vi "S2C_STEP_ShowMenu.vi"(8 "Error In":errorcluster, 9 "Cell Position":T1, 10 "MenuRef":refnum<k9>, 11 "CtlRef":refnum<vi>) -> (0 "Error Out":errorcluster, 3 "Discard?":bool)   [LabVIEW 2015]
doc: "Loads the popup menu for the selected Fornax command parameter."
uses:
  <vilib>/Utility/miscctls.llb/LVRowAndColumnTypeDef.ctl
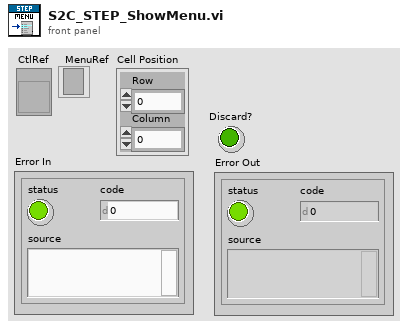
[diagram p1: front panel]
types:
  T1 = typedef "LVRowAndColumnTypeDef.ctl" = cluster{"Row":i32, "Column":i32}
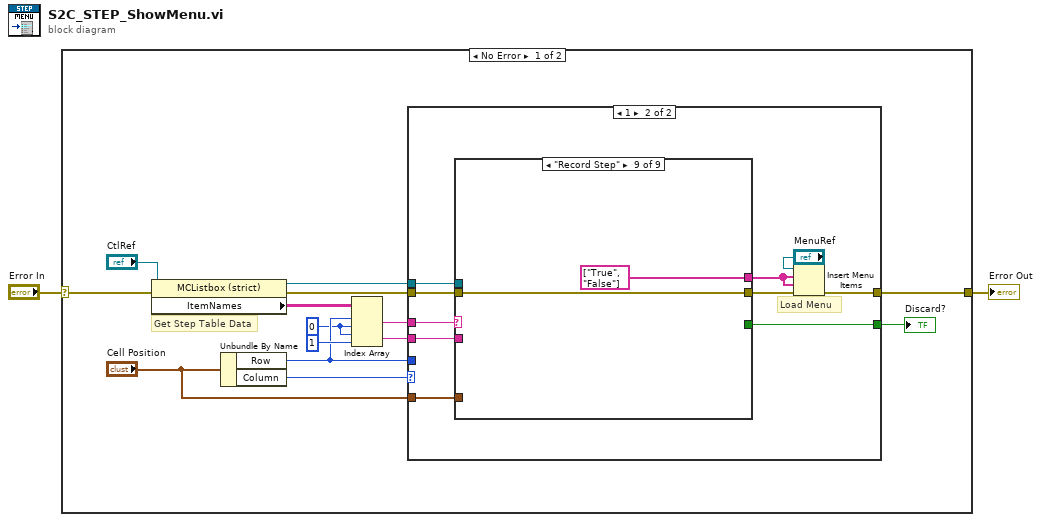
[diagram p0: block diagram]
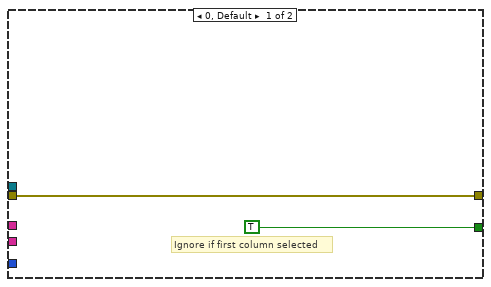
[diagram p2: hidden frame]
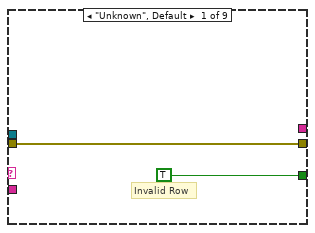
[diagram p3: hidden frame]
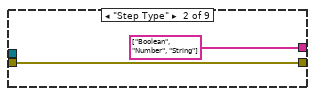
[diagram p4: hidden frame]
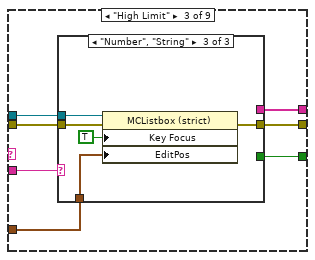
[diagram p5: hidden frame]
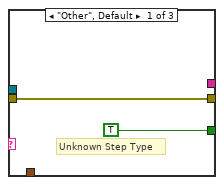
[diagram p6: hidden frame]
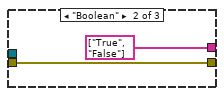
[diagram p7: hidden frame]
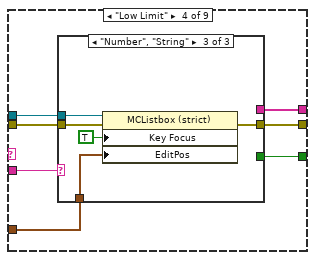
[diagram p8: hidden frame]
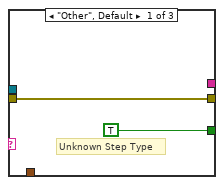
[diagram p9: hidden frame]
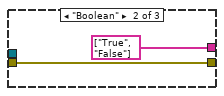
[diagram p10: hidden frame]
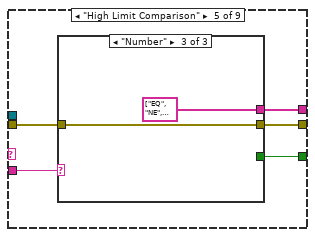
[diagram p11: hidden frame]
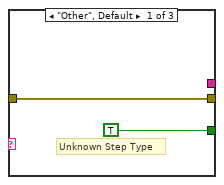
[diagram p12: hidden frame]
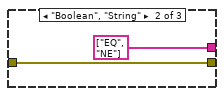
[diagram p13: hidden frame]
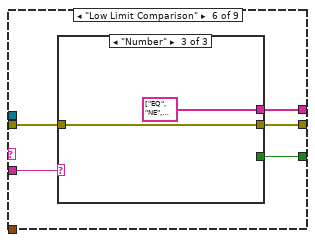
[diagram p14: hidden frame]
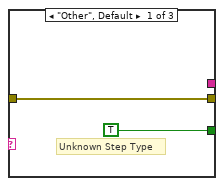
[diagram p15: hidden frame]
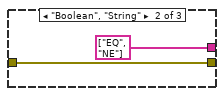
[diagram p16: hidden frame]
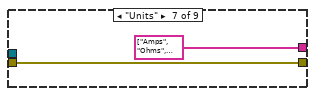
[diagram p17: hidden frame]
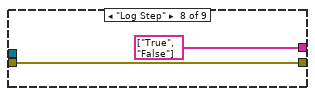
[diagram p18: hidden frame]
diagram:
  n1 = case shown="No Error" "Error In" {
    selector: "Error In" -> [w11 w93]
    tunnel: [w16 w93] -> w1
    frame No Error {
      w3 = 0 ("disabled index (col)")
      # "Get Step Table Data"
      n2 = property class="MCListbox (strict)"(reference="CtlRef", error in=w11) -> (reference out=w8:refnum<vi>, error out=w9:errorcluster, "ItemNames"=w7:string[][])
      n3 = Unbundle By Name("Cell Position") -> ("Row"=w6:i32, "Column"=w13:i32)
      n4 = Index Array(array=w7, index (row) #1=w6, index (col) #1=w3, index (row) #2=w3, index (col) #2=1 ("index (col)")) -> (element #1=w5:string, element #2=w4:string)
      n5 = case shown="1" w13 {
        tunnel: w9 -> [w18 w28]
        tunnel: [w18 w27] -> w16
        tunnel: w6 -> [_ _]
        tunnel: [TRUE w26] -> w15
        tunnel: "Cell Position" -> [_ w25]
        tunnel: w8 -> [_ w24]
        tunnel: w5 -> [_ w20]
        tunnel: w4 -> [_ w19]
        frame 0, Default {
          # "Ignore if first column selected"
        }
        frame 1 {
          # "Load Menu"
          n6 = case shown="\"Record Step\"" w20 {
            tunnel: w28 -> [w30 w32 w34 w51 w65 w76 w88 w90 w92]
            tunnel: [w30 w32 w39 w55 w69 w80 w88 w90 w92] -> w21
            tunnel: w24 -> [_ _ w33 w50 _ _ _ _ _]
            tunnel: w25 -> [_ _ w38 w54 _ _ _ _ _]
            tunnel: [TRUE _ w36 w53 w67 w78 _ _ _] -> w26
            tunnel: [_ string[] ["Boolean", "Number", "String"] w37 w49 w68 w79 string[] ["Amps", "Ohms", "Watts", "Volts", "None", "Other"] string[] ["True", "False"] string[] ["True", "False"]] -> w22
            tunnel: w19 -> [_ _ w35 w52 w66 w77 _ _ _]
            frame "Unknown", Default {
              # "Invalid Row"
            }
            frame "Step Type" {
            }
            frame "High Limit" {
              n7 = case shown="\"Number\", \"String\"" w35 {
                tunnel: [w41 w42 w46] -> w39
                tunnel: w34 -> [w41 w42 w47]
                tunnel: w33 -> [_ _ w48]
                tunnel: w38 -> [_ _ w44]
                tunnel: [_ string[] ["True", "False"] _] -> w37
                tunnel: [TRUE _ _] -> w36
                frame "Other", Default {
                  # "Unknown Step Type"
                }
                frame "Boolean" {
                }
                frame "Number", "String" {
                  n8 = property class="MCListbox (strict)"(reference=w48, error in=w47, "Key Focus"=TRUE, "EditPos"=w44) -> (error out=w46:errorcluster)  [unwired: 1 out]
                }
              }
            }
            frame "Low Limit" {
              n9 = case shown="\"Number\", \"String\"" w52 {
                tunnel: [w57 w58 w62] -> w55
                tunnel: w51 -> [w57 w58 w63]
                tunnel: w50 -> [_ _ w64]
                tunnel: w54 -> [_ _ w60]
                tunnel: [TRUE _ _] -> w53
                tunnel: [_ string[] ["True", "False"] _] -> w49
                frame "Other", Default {
                  # "Unknown Step Type"
                }
                frame "Boolean" {
                }
                frame "Number", "String" {
                  n10 = property class="MCListbox (strict)"(reference=w64, error in=w63, "Key Focus"=TRUE, "EditPos"=w60) -> (error out=w62:errorcluster)  [unwired: 1 out]
                }
              }
            }
            frame "High Limit Comparison" {
              n11 = case shown="\"Number\"" w66 {
                tunnel: [w71 w73 w75] -> w69
                tunnel: w65 -> [w71 w73 w75]
                tunnel: [_ string[] ["EQ", "NE"] string[] ["EQ", "NE", "LT", "LE"]] -> w68
                tunnel: [TRUE _ _] -> w67
                frame "Other", Default {
                  # "Unknown Step Type"
                }
                frame "Boolean", "String" {
                }
                frame "Number" {
                }
              }
            }
            frame "Low Limit Comparison" {
              n12 = case shown="\"Number\"" w77 {
                tunnel: [w82 w83 w86] -> w80
                tunnel: w76 -> [w82 w83 w86]
                tunnel: [_ string[] ["EQ", "NE"] string[] ["EQ", "NE", "GT", "GE"]] -> w79
                tunnel: [TRUE _ _] -> w78
                frame "Other", Default {
                  # "Unknown Step Type"
                }
                frame "Boolean", "String" {
                }
                frame "Number" {
                }
              }
            }
            frame "Units" {
            }
            frame "Log Step" {
            }
            frame "Record Step" {
            }
          }
          n13 = Insert Menu Items(6:w21, 7:w22, 8:w22, 9:"MenuRef") -> (0:w27:errorcluster)  [unwired: 2 in, 2 out]
        }
      }
      "Discard?" <- w15
    }
    frame Error {
    }
  }
  "Error Out" <- w1
